vi "Type Signal loaded form database.vi"(8 "error in":errorcluster, 9 "Nombre de la Prueba":string, 10 "Digital Signal":T1={"DAQ Board Name"="DAQ_Simu1", "Port Digitales"=[], "rate"=1000.0, "Tiempo"=100}, 11 "Type Signal":T2={"DAQ Board Name"="DAQ_Simu1", "Analogicos Canales"=["DAQ_Simu1/ai1", "DAQ_Simu1/ai2"], "rate"=1000.0, "number of samples "=1000, "Tiempo"=100}) -> (0 "error out":errorcluster)   [LabVIEW 2020, in "Settings.lvlib"]
doc: "Type signal was loaded from database\n_____\nCreated using Delacor QMH Event Scripter 6.0.0.121."
uses:
  Settings.lvlib
  typeSignal--cluster.ctl
  Digital typeSignal--cluster.ctl
  Type Signal loaded form database Argument--cluster.ctl
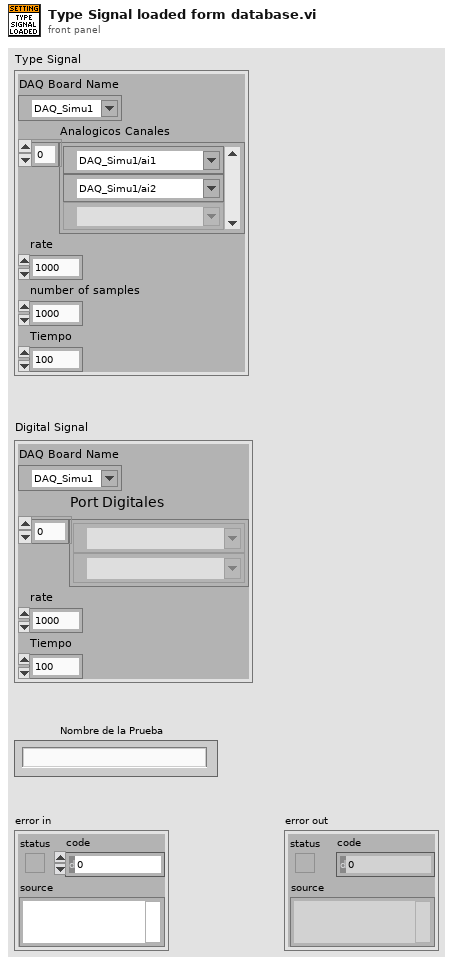
[diagram p1: front panel]
types:
  T1 = typedef "Digital typeSignal--cluster.ctl" = cluster{"DAQ Board Name":tag, "Port Digitales":tag[], "rate":dbl, "Tiempo":i32}
  T2 = typedef "typeSignal--cluster.ctl" = cluster{"DAQ Board Name":tag, "Analogicos Canales":tag[], "rate":dbl, "number of samples ":i32, "Tiempo":i32}
  T3 = typedef "Settings.lvlib/Type Signal loaded form database Argument--cluster.ctl" = cluster{"Type Signal":T2, "Digital Signal":T1, "Nombre de la Prueba":string}
  T4 = typedef "Settings.lvlib/Request Events--cluster.ctl" = cluster{"Stop Module":refnum<user-event>, "Show Panel":refnum<user-event>, "Hide Panel":refnum<user-event>, "Get Module Execution Status":refnum<user-event>, "Show Diagram":refnum<user-event>, "Add signal":refnum<user-event>, "Delete table":refnum<user-event>, "Cancel":refnum<user-event>, "Type Signal loaded form database":refnum<user-event>, "Delete All Table":refnum<user-event>, "Add Digital Signal":refnum<user-event>, "Delete Digital table":refnum<user-event>, "Complete Tarea":refnum<user-event>}
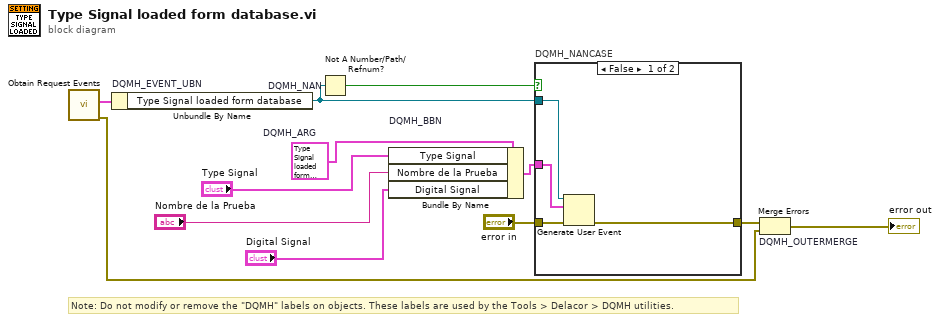
[diagram p0: block diagram]
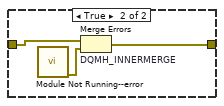
[diagram p2: hidden frame]
diagram:
  w6 = T3 {"Type Signal"={"DAQ Board Name"="DAQ_Simu1", "Analogicos Canales"=["DAQ_Simu1/ai1", "DAQ_Simu1/ai2"], "rate"=1000.0, "number of samples "=1000, "Tiempo"=100}, "Digital Signal"={"DAQ Board Name"="DAQ_Simu1", "Port Digitales"=[], "rate"=1000.0, "Tiempo"=100}, "Nombre de la Prueba"=""}  # DQMH_ARG
  # "Note: Do not modify or remove the \"DQMH\" labels on objects. These labels are used by the Tools > Delacor > DQMH utilities."
  n1 = call "Obtain Request Events.vi"() -> ("error out"=w3:errorcluster, "Settings Request Events"=w2:T4)  [unwired: 10 in]
  n2 = Unbundle By Name "DQMH_EVENT_UBN"(w2) -> ("Type Signal loaded form database"=w8:refnum<user-event>)
  n3 = Not A Number/Path/Refnum? "DQMH_NAN"(number/path/refnum=w8) -> (NaN/Path/Refnum?=w9:bool)
  n4 = Bundle By Name "DQMH_BBN"(cluster=w6, "Type Signal"="Type Signal", "Nombre de la Prueba"="Nombre de la Prueba", "Digital Signal"="Digital Signal") -> (w10:T3)
  n5 = case "DQMH_NANCASE" shown="False" w9 {
    tunnel: "error in" -> [w16 w19]
    tunnel: [w15 w18] -> w7
    tunnel: w8 -> [w14 _]
    tunnel: w10 -> [w13 _]
    frame False {
      n6 = Generate User Event(user event=w14, event data cluster=w13, error in=w16) -> (error out=w15:errorcluster)  [unwired: 1 in, 1 out]
    }
    frame True {
      n7 = call "Module Not Running--error.vi"() -> ("error out"=w17:errorcluster)  [unwired: 11 in]
      n8 = Merge Errors "DQMH_INNERMERGE"(w19, w17) -> (w18:errorcluster)
    }
  }
  n9 = Merge Errors "DQMH_OUTERMERGE"(w7, w3) -> (→"error out":errorcluster)
